vi "ReadChannels.vi"(8 "error in":errorcluster, 9 "Data in":sgl[](array[numeric]), 10 "number of channels":u16, 11 "Modbus master in":refnum<class "Modbus Master.lvclass">) -> (0 "error out":errorcluster, 2 "Data out":sgl[](array[numeric]), 3 "Modbus master out":refnum<class "Modbus Master.lvclass">)   [LabVIEW 2016]
doc: "Get data channel from DAS240 using Modbus TCP. Give the number of channels wanted, and read on TCP will be iterated each 62 channels read."
uses:
  <vilib>/NI/Modbus Library/API/Master/Modbus Master.lvclass
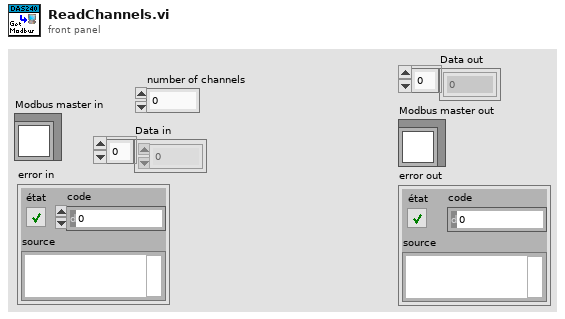
[diagram p1: front panel]
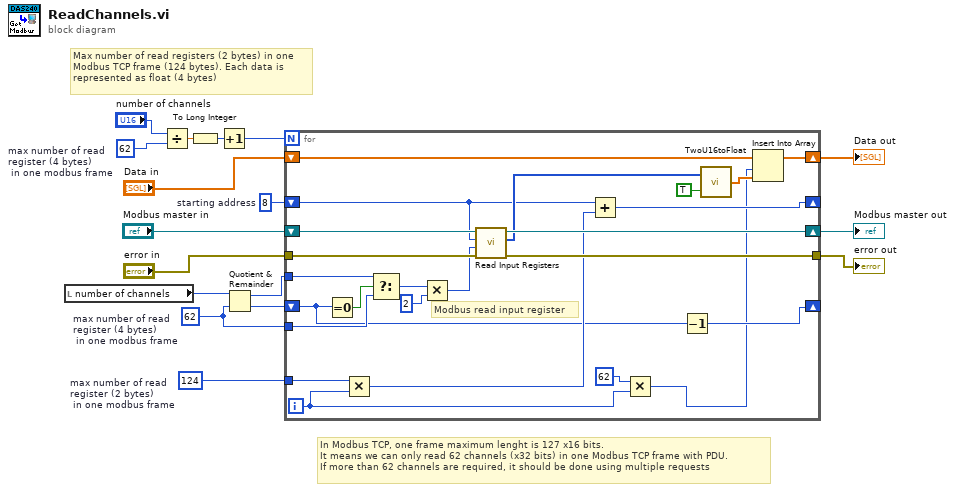
[diagram p0: block diagram]
diagram:
  w4 = u16 62  # max number of read register (4 bytes)  in one modbus frame
  w8 = 124  # max number of read register (2 bytes)  in one modbus frame
  w10 = u16 62  # max number of read register (4 bytes)  in one modbus frame
  w17 = 8  # starting address
  # "In Modbus TCP, one frame maximum lenght is 127 x16 bits. \nIt means we can only read 62 channels (x32 bits) in one Modbus TCP frame with PDU.\nIf more than 62 channels are required, it should be done using multiple requests"
  # "Max number of read registers (2 bytes) in one\nModbus TCP frame (124 bytes). Each data is\nrepresented as float (4 bytes)"
  n1 = local read "number of channels"() -> (w7:u16)
  n2 = Divide(x="number of channels", y=w10) -> (x/y=w16:dbl)
  n3 = To Long Integer(number=w16) -> (32bit integer=w15:i32)
  n4 = Increment(x=w15) -> (x+1=w14:i32)
  n5 = Quotient & Remainder(x=w7, y=w4) -> (x-y*floor(x/y)=w5:u16, floor(x/y)=w6:u16)
  n6 = for {
    N: w14 -> [_]
    tunnel: "error in" -> [w40]
    tunnel: [w38] -> w1
    shift-right: [w36] -> _
    shift-left: w17 -> [w30]
    tunnel: w8 -> [w37]
    shift-right: [w31] -> w3
    shift-left: "Data in" -> [w33]
    shift-right: [w39] -> w2
    shift-left: "Modbus master in" -> [w41]
    shift-right: [w21] -> _
    shift-left: w6 -> [w22]
    tunnel: w5 -> [w27]
    tunnel: w4 -> [w26]
    i -> [w19]
    # "Modbus read input register"
    n7 = Equal To 0?(x=w22) -> (x = 0?=w28:bool)
    n8 = Multiply(x=w37, y=w19) -> (x*y=w29:i32)
    n9 = Select(t=w27, s=w28, f=w26) -> (s? t:f=w25:u16)
    n10 = Multiply(x=w25, y=u16 2) -> (x*y=w23:u16)
    n11 = call-dynamic "Read Input Registers.vi"("error in"=w40, "number of inputs"=w23, "starting address"=w30, "Modbus master in"=w41) -> ("error out"=w38:errorcluster, "register values"=w35:u16[], "Modbus master out"=w39:refnum<class "Modbus Master.lvclass">)  [unwired: 5 in]
    n12 = Add(x=w30, y=w29) -> (x+y=w36:i32)
    n13 = Multiply(x=62, y=w19) -> (x*y=w18:i32)
    n14 = Decrement(x=w22) -> (x-1=w21:u16)
    n15 = call "TwoU16toFloat.vi"("LittleEndian? (F)"=TRUE, "Register Array"=w35) -> ("Converted Array"=w32:sgl[])
    n16 = Insert Into Array(array=w33, index=w18, new element=w32) -> (w31:sgl[])
  }
  "Data out" <- w3
  "Modbus master out" <- w2
  "error out" <- w1
